vi "Actor Core.vi"(8 "error in":errorcluster, 11 "Integrate in":refnum<class "Integrate.lvclass">) -> (0 "error out":errorcluster, 3 "Actor out":refnum<class "Actor.lvclass">)   [LabVIEW 2018, in "Integrate.lvclass"]
doc: "(<B>Filename</B>: Actor Framework.lvlib:Actor.lvclass:Actor Core.vi)\n\nReceives messages to the actor, reacts to them, and initiates any error handling that may shut the actor down.\n\nDescendant classes may override this VI to append parallel tasks for the actor to complete while it handles messages. Overrides use the Call Parent Method node."
uses:
  Integrate.lvclass
  C:/github/LabActor/Template Module/Template Module.lvclass
  C:/Program Files/National Instruments/LabVIEW 2018/vi.lib/ActorFramework/Actor/Actor.lvclass
  <vilib>/ActorFramework/Actor/Actor.lvclass
  Integrator Configuration.ctl
  NHMFL_Core/Libraries/Utilities/Controls/Integrate channel.ctl
  Channel peak.ctl
  Template Module/Template Module.lvclass/Template Module.ctl
  <vilib>/ActorFramework/Actor/Actor.lvclass/Actor.ctl
  <vilib>/ActorFramework/Message Enqueuer/Message Enqueuer.lvclass/Message Enqueuer.ctl
  NHMFL_Core/Libraries/Instruments/Results/File Path Result/File Path Result.lvclass
  C:/github/NHMFL_Core/Libraries/Instruments/Results/Acquired Result/Acquired Result.lvclass
  Process Object Messages/Process Result Msg/Process Result Msg.lvclass/Process Result Msg.ctl
  Template Module/Read stop event.vi
  <vilib>/ActorFramework/Message Enqueuer/Init from Existing Queue.vi
  <vilib>/ActorFramework/Message Enqueuer/Enqueue.vi
  Process Object Messages/Process Result Msg/Process Result Msg.lvclass
  C:/Program Files/National Instruments/LabVIEW 2018/vi.lib/ActorFramework/Message/Message.lvclass
  <vilib>/ActorFramework/Message Priority Queue/Priority Enqueue.vi
  Process Object/Process Object.lvclass
  <vilib>/ActorFramework/Message Enqueuer/Message Enqueuer.lvclass
panel:
  in  "Re-process":bool
  in  "Input file":path
  out "Channel peaks":T1[](array[typedef]) {"Peak" format="%#_4p"}
  out "Name":string
  in  "Configuration":T2={"Integrate"=[{"Channel"="Bdot", "Output name"="Field", "Factor"=1.0, "Start time"=nan, "Duration"=nan, "Fix drift"=FALSE}], "Offset duration "=0.0095, "TDMS group name"="p"} {"Offset duration" format="%#_6ps"; "Integrate"."Duration" format="%#_6ps"; "Integrate"."Start time" format="%#_6ps"}
  # "Input CH"
  # "X-Factor"
  # "Output CH"
  # "Start"
  # "Duration"
  # "Fix drift"
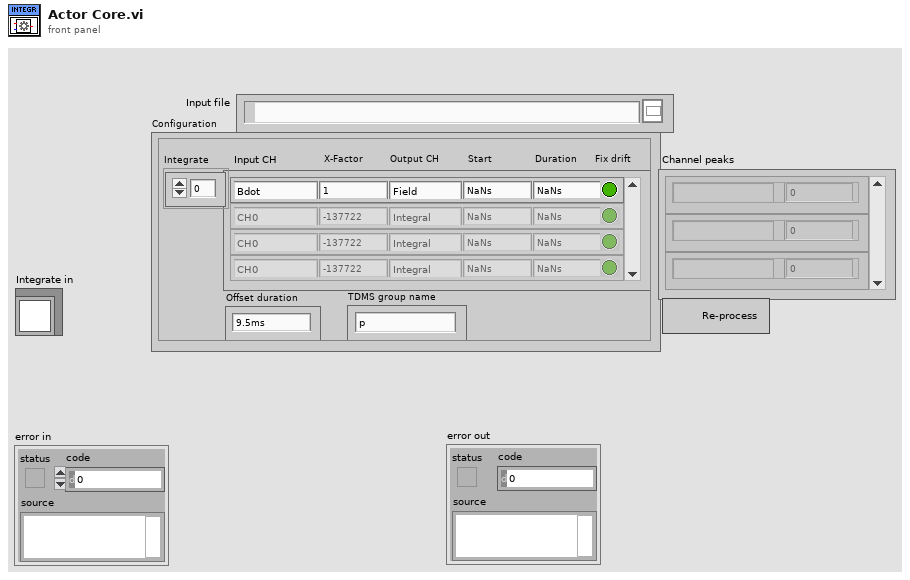
[diagram p1: front panel]
types:
  T1 = typedef "Channel peak.ctl" = cluster{"Peak":dbl, "Name":string}
  T2 = typedef "Integrator Configuration.ctl" = cluster{"Integrate":T3[], "Offset duration ":dbl, "TDMS group name":string}
  T3 = typedef "Integrate channel.ctl" = cluster{"Channel":string, "Output name":string, "Factor":dbl, "Start time":dbl, "Duration":dbl, "Fix drift":bool}
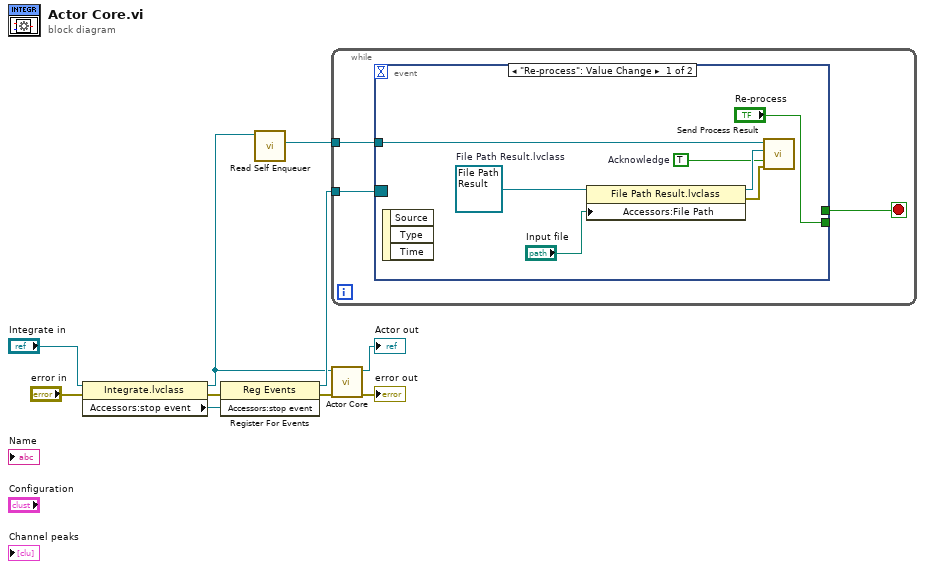
[diagram p0: block diagram]
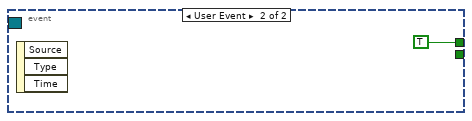
[diagram p2: hidden frame]
diagram:
  n1 = property class="Integrate.lvclass"(reference="Integrate in", error in="error in") -> (reference out=w2:refnum<class "Integrate.lvclass">, error out=w6:errorcluster, "Accessors:stop event"=w8:refnum<user-event>)
  n2 = register-events(error in=w6, w8) -> (reference out=w7:refnum<event-registration>, error out=w1:errorcluster)  [unwired: 1 in]
  n3 = call <vilib>:"Read Self Enqueuer.vi"("Actor"=w2) -> ("Self Enqueuer"=w5:refnum<class "Message Enqueuer.lvclass">)  [unwired: 10 in]
  n4 = while {
    tunnel: w7 -> [w13]
    tunnel: w5 -> [w11]
    stop <- w12 stop-if-true
    n5 = event shown="[0] \"Re-process\": Value Change" {
      selector: w13 -> [_ _]
      dyn-events: _ -> [_ _]
      timeout: _ -> [_ _]
      tunnel: [_ TRUE] -> w12
      tunnel: w11 -> [w20 _]
      tunnel: ["Re-process" _] -> _
      event "Re-process": Value Change {
        w14 = TRUE  # Acknowledge
        w19 = refnum<class "File Path Result.lvclass"> refnum  # File Path Result.lvclass
        n6 = event-data() -> ()  [unwired: 1 in, 3 out]
        n7 = property class="File Path Result.lvclass"(reference=w19, "Accessors:File Path"="Input file") -> (reference out=w18:refnum<class "File Path Result.lvclass">, error out=w17:errorcluster)  [unwired: 1 in]
        n8 = call "Send Process Result.vi"("error in (no error)"=w17, "Acknowledge"=w14, "Result in"=w18, "Message Enqueuer"=w20) -> ()  [unwired: 6 in, 2 out]
      }
      event User Event {
        n9 = event-data() -> ()  [unwired: 1 in, 3 out]
      }
    }
  }
  n10 = call-parent "Actor Core.vi"("error in"=w1, "Measure Object in"=w2) -> ("error out"=→"error out":errorcluster, "Actor out"=→"Actor out":refnum<class "Actor.lvclass">)  [unwired: 8 in]
